vi "SV Measure Delay (Equal Polarity).vi"(0 "reference signal":waveform(dbl), 1 "ignore time stamp (T)":bool=TRUE, 5 "delayed signal":waveform(dbl), 7 "method":u16(ring)=1 items=["Trigger", "Cross correlation", "Phase lag"], 11 "error in":errorcluster, 12 "trigger parameters":T1={"level"=0.0, "slope"=0, "hysteresis"=-0.1} {"hysteresis" format="%.2p"; "slope" items=["Falling", "Rising"]; "level" format="%.2p"}) -> (4 "delay [s]":dbl format="%_4p", 6 "delay [samples]":dbl format="%_4f", 15 "error out":errorcluster)   [LabVIEW 2017, in "SoundVib_Calibration.lvlib"]
doc: "Use this VI to measure the propagation delay of a response signal. Use this VI when performing stimulus-response measurements to polarity normalize and time align the response signals prior to precision block processing. Use the equal polarity instance when the delayed signal exhibits equal polarity and simple time delay."
uses:
  <vilib>/addons/Sound and Vibration/svt_Calibration/SoundVib_Calibration.lvlib
  <vilib>/addons/_NISVFA/_Shared subVIs/Controls/svc_Analog Level Trigger Configuration.ctl
  <vilib>/Analysis/baseanly.llb/Mean (DBL).vi
  <vilib>/measure/matone.llb/Extract Single Tone Information 1 Chan.vi
  <vilib>/Analysis/2dsp.llb/1D Cross Correlation (DBL).vi
  <vilib>/measure/mamon.llb/Trigger Detection for 1 Channel.vi
  <vilib>/Analysis/NI_AALPro.lvlib
  <vilib>/measure/NI_MAPro.lvlib
  <vilib>/Analysis/NI_AAL_SigProc.lvlib
  <vilib>/Analysis/NI_AALBase.lvlib
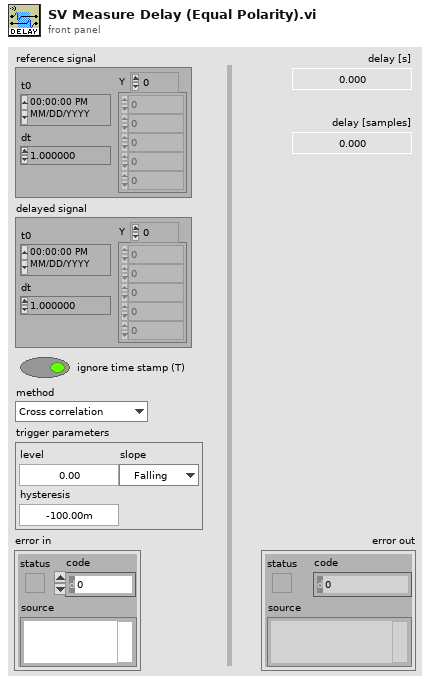
[diagram p1: front panel]
types:
  T1 = typedef "svc_Analog Level Trigger Configuration.ctl" = cluster{"level":dbl, "slope":u16, "hysteresis":dbl}
  T2 = cluster{"approx freq. (optional)":dbl, "search (+/- % of Fsampl.)":dbl}
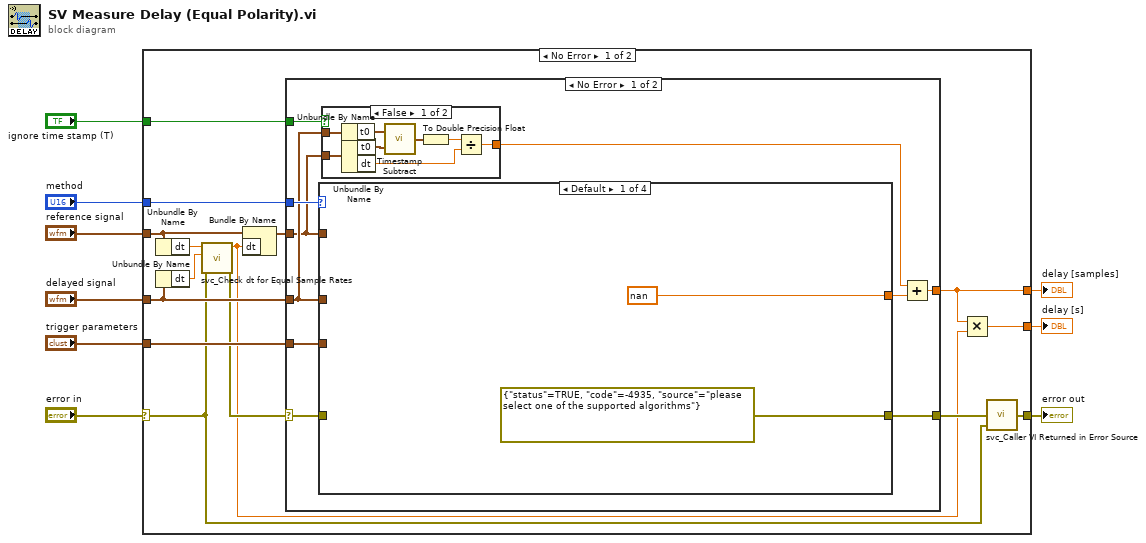
[diagram p0: block diagram]
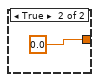
[diagram p2: hidden frame]
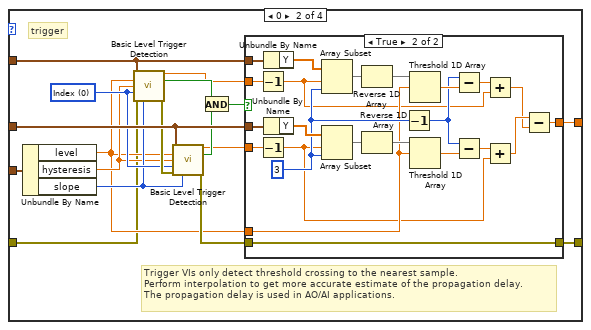
[diagram p3: hidden frame]
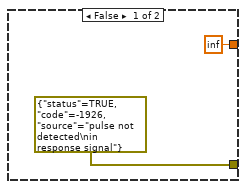
[diagram p4: hidden frame]
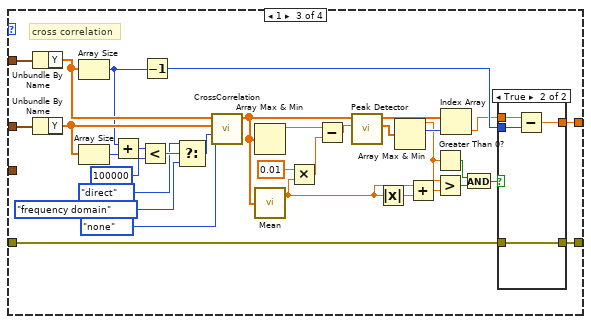
[diagram p5: hidden frame]
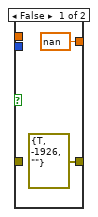
[diagram p6: hidden frame]
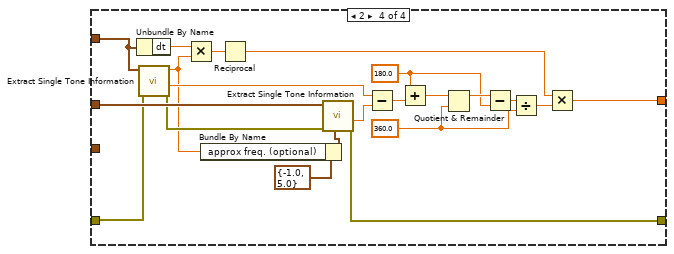
[diagram p7: hidden frame]
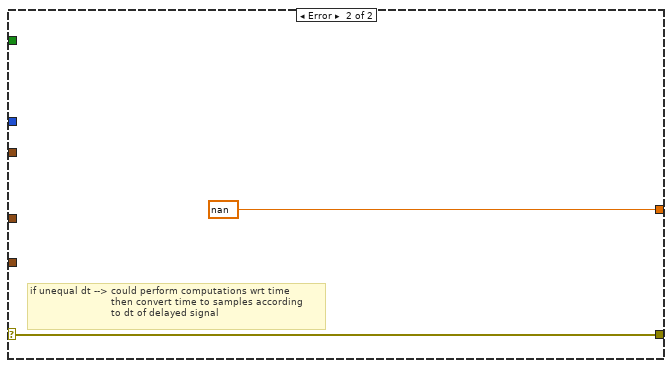
[diagram p8: hidden frame]
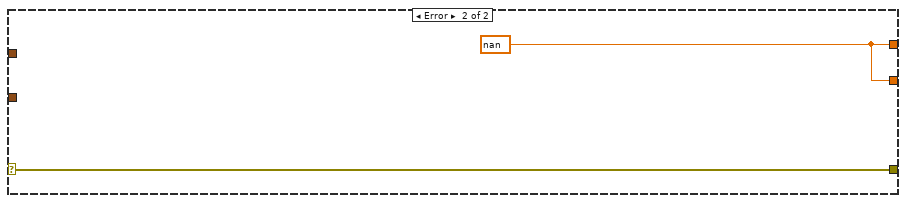
[diagram p9: hidden frame]
diagram:
  n1 = case shown="No Error" "error in" {
    selector: "error in" -> [w16 w151]
    tunnel: "method" -> [w24 _]
    tunnel: "trigger parameters" -> [w23 _]
    tunnel: [w17 w151] -> w7
    tunnel: "delayed signal" -> [w20 _]
    tunnel: "reference signal" -> [w14 _]
    tunnel: "ignore time stamp (T)" -> [w21 _]
    tunnel: [w12 w150] -> w3
    tunnel: [w10 w150] -> w1
    frame No Error {
      n2 = Unbundle By Name(w14) -> ("dt"=w19:dbl)
      n3 = Unbundle By Name(w20) -> ("dt"=w18:dbl)
      n4 = call <vilib>:"svc_Check dt for Equal Sample Rates.vi"("error in (no error)"=w16, "dt Y"=w18, "dt X"=w19) -> ("error out"=w15:errorcluster, "dt Y"=w11:dbl)  [unwired: 7 in]
      n5 = Bundle By Name(cluster=w14, "dt"=w11) -> (w13:waveform(dbl))
      n6 = case shown="No Error" w15 {
        selector: w15 -> [w26 w149]
        tunnel: w24 -> [w34 _]
        tunnel: w23 -> [w33 _]
        tunnel: [w32 w149] -> w22
        tunnel: w21 -> [w31 _]
        tunnel: [w30 nan] -> w12
        tunnel: w20 -> [w27 _]
        tunnel: w13 -> [w25 _]
        frame No Error {
          n7 = case shown="Default" w34 {
            tunnel: w27 -> [_ w62 w98 w147]
            tunnel: w25 -> [_ w61 w100 w140]
            tunnel: [nan w60 w117 w135] -> w29
            tunnel: w33 -> [_ w51 _ _]
            tunnel: w26 -> [_ w47 w101 w146]
            tunnel: [errorcluster {"status"=TRUE, "code"=-4935, "source"="please select one of the supported algorithms"} ("error out") w46 w115 w131] -> w32
            frame Default {
            }
            frame 0 {
              w52 = u16 0 items=["Index", "Time"] ("mode")
              # "trigger"
              # "Trigger VIs only detect threshold crossing to the nearest sample. \nPerform interpolation to get more accurate estimate of the propagation delay.\nThe propagation delay is used in AO/AI applications."
              n8 = Unbundle By Name(w51) -> ("level"=w48:dbl, "hysteresis"=w49:dbl, "slope"=w50:u16)
              n9 = call-poly <vilib>:"Basic Level Trigger Detection.vi"("signal in"=w61, "level"=w48, "hysteresis"=w49, "location mode"=w52, "error in (no error)"=w47, "trigger slope"=w50) -> ("trigger location"=w54:dbl, "trigger detected?"=w59:bool, "error out"=w57:errorcluster)  [unwired: 7 in]
              n10 = call-poly <vilib>:"Basic Level Trigger Detection.vi"("signal in"=w62, "level"=w48, "hysteresis"=w49, "location mode"=w52, "error in (no error)"=w57, "trigger slope"=w50) -> ("trigger location"=w55:dbl, "trigger detected?"=w58:bool, "error out"=w56:errorcluster)  [unwired: 7 in]
              n11 = And(x=w59, y=w58) -> (x .and. y?=w53:bool)
              n12 = case shown="True" w53 {
                tunnel: w55 -> [_ w72]
                tunnel: w54 -> [_ w84]
                tunnel: [inf w87] -> w60
                tunnel: w56 -> [_ w86]
                tunnel: [errorcluster {"status"=TRUE, "code"=-1926, "source"="pulse not detected\nin response signal"} ("error out") w86] -> w46
                tunnel: w61 -> [_ w85]
                tunnel: w48 -> [_ w71]
                tunnel: w62 -> [_ w76]
                frame False {
                }
                frame True {
                  w73 = 3 ("length")
                  n13 = Decrement(x=w84) -> (x-1=w68:dbl)
                  n14 = Decrement(x=w72) -> (x-1=w67:dbl)
                  n15 = Unbundle By Name(w85) -> ("Y"=w83:dbl[])
                  n16 = Unbundle By Name(w76) -> ("Y"=w75:dbl[])
                  n17 = Array Subset(array=w83, index=w68, length=w73) -> (w82:dbl[])
                  n18 = Array Subset(array=w75, index=w67, length=w73) -> (w77:dbl[])
                  n19 = Reverse 1D Array(array=w82) -> (reversed array=w81:dbl[])
                  n20 = Reverse 1D Array(array=w77) -> (reversed array=w78:dbl[])
                  n21 = Decrement(x=w73) -> (x-1=w74:i32)
                  n22 = Threshold 1D Array(2:w71, 3:w81) -> (0:w80:dbl)  [unwired: 1 in]
                  n23 = Threshold 1D Array(2:w71, 3:w78) -> (0:w79:dbl)  [unwired: 1 in]
                  n24 = Subtract(x=w74, y=w80) -> (x-y=w69:dbl)
                  n25 = Subtract(x=w74, y=w79) -> (x-y=w70:dbl)
                  n26 = Add(x=w69, y=w68) -> (x+y=w65:dbl)
                  n27 = Add(x=w70, y=w67) -> (x+y=w66:dbl)
                  n28 = Subtract(x=w66, y=w65) -> (x-y=w87:dbl)
                }
              }
            }
            frame 1 {
              # "cross correlation"
              n29 = Unbundle By Name(w100) -> ("Y"=w99:dbl[])
              n30 = Unbundle By Name(w98) -> ("Y"=w97:dbl[])
              n31 = Array Size(array=w99) -> (size(s)=w96:i32)
              n32 = Array Size(array=w97) -> (size(s)=w95:i32)
              n33 = Add(x=w96, y=w95) -> (x+y=w94:i32)
              n34 = Less?(x=w94, y=100000) -> (x < y?=w92:bool)
              n35 = Decrement(x=w96) -> (x-1=w116:i32)
              n36 = Select(t=enum32{"direct", "frequency domain"}."direct" ("algorithm"), s=w92, f=enum32{"direct", "frequency domain"}."frequency domain" ("algorithm")) -> (s? t:f=w89:enum32{"direct", "frequency domain"})
              n37 = call-poly <vilib>:"CrossCorrelation.vi"("normalization"=enum32{"none", "unbiased", "biased"}."none", "algorithm"=w89, "Y"=w97, "X"=w99) -> ("Rxy"=w111:dbl[])  [unwired: 6 in, 1 out]
              n38 = Array Max & Min(array=w111) -> (max value=w120:dbl)  [unwired: 3 out]
              n39 = call-poly <vilib>:"Mean.vi"("X"=w111) -> ("mean"=w104:dbl)  [unwired: 1 out]
              n40 = Multiply(x=0.01, y=w104) -> (x*y=w103:dbl)
              n41 = Subtract(x=w120, y=w103) -> (x-y=w119:dbl)
              n42 = call <vilib>:"Peak Detector.vi"("threshold"=w119, "X"=w111) -> ("Amplitudes"=w118:dbl[], "Locations"=w114:dbl[])  [unwired: 5 in, 3 out]
              n43 = Absolute Value(x=w104) -> (abs(x)=w109:dbl)
              n44 = Array Max & Min(array=w118) -> (max value=w106:dbl, max index (indices)=w113:i32)  [unwired: 2 out]
              n45 = Add(x=w104, y=w109) -> (x+y=w110:dbl)
              n46 = Greater Than 0?(x=w106) -> (x > 0?=w105:bool)
              n47 = Greater?(x=w106, y=w110) -> (0:w107:bool)
              n48 = Index Array(array=w114, index=w113) -> (element=w112:dbl)
              n49 = And(x=w105, y=w107) -> (x .and. y?=w108:bool)
              n50 = case shown="True" w108 {
                tunnel: [nan w126] -> w117
                tunnel: w116 -> [_ w125]
                tunnel: w101 -> [_ w124]
                tunnel: [errorcluster {"status"=TRUE, "code"=-1926, "source"=""} ("error out") w124] -> w115
                tunnel: w112 -> [_ w123]
                frame False {
                }
                frame True {
                  n51 = Subtract(x=w123, y=w125) -> (x-y=w126:dbl)
                }
              }
            }
            frame 2 {
              w127 = 180.0 ("y")
              w133 = 360.0 ("y")
              n52 = Unbundle By Name(w140) -> ("dt"=w139:dbl)
              n53 = call-poly <vilib>:"Extract Single Tone Information.vi"("error in (no error)"=w146, "time signal in"=w140) -> ("error out"=w145:errorcluster, "detected phase (deg)"=w142:dbl, "detected frequency"=w138:dbl)  [unwired: 4 in, 3 out]
              n54 = Multiply(x=w139, y=w138) -> (x*y=w136:dbl)
              n55 = Bundle By Name(cluster=T2 {"approx freq. (optional)"=-1.0, "search (+/- % of Fsampl.)"=5.0} ("advanced search"), "approx freq. (optional)"=w138) -> (w143:T2)
              n56 = Reciprocal(x=w136) -> (1/x=w132:dbl)
              n57 = call-poly <vilib>:"Extract Single Tone Information.vi"("advanced search"=w143, "error in (no error)"=w145, "time signal in"=w147) -> ("error out"=w131:errorcluster, "detected phase (deg)"=w141:dbl)  [unwired: 3 in, 4 out]
              n58 = Subtract(x=w142, y=w141) -> (x-y=w128:dbl)
              n59 = Add(x=w127, y=w128) -> (x+y=w130:dbl)
              n60 = Quotient & Remainder(x=w130, y=w133) -> (x-y*floor(x/y)=w137:dbl)  [unwired: 1 out]
              n61 = Subtract(x=w137, y=w127) -> (x-y=w129:dbl)
              n62 = Divide(x=w129, y=w133) -> (x/y=w134:dbl)
              n63 = Multiply(x=w132, y=w134) -> (x*y=w135:dbl)
            }
          }
          n64 = case shown="False" w31 {
            tunnel: w27 -> [w42 _]
            tunnel: w25 -> [w41 _]
            tunnel: [w36 0.0] -> w28
            frame False {
              n65 = Unbundle By Name(w42) -> ("t0"=w40:timestamp)
              n66 = Unbundle By Name(w41) -> ("t0"=w39:timestamp, "dt"=w35:dbl)
              n67 = call <vilib>:"Timestamp Subtract.vi"("y"=w39, "x"=w40) -> ("x - y"=w38:timestamp)
              n68 = To Double Precision Float(number=w38) -> (double precision float=w37:dbl)
              n69 = Divide(x=w37, y=w35) -> (x/y=w36:dbl)
            }
            frame True {
            }
          }
          n70 = Add(x=w28, y=w29) -> (x+y=w30:dbl)
        }
        frame Error {
          # "if unequal dt --> could perform computations wrt time \n                           then convert time to samples according\n                           to dt of delayed signal"
        }
      }
      n71 = Multiply(x=w12, y=w11) -> (x*y=w10:dbl)
      n72 = call <vilib>:"svc_Caller VI Returned in Error Source.vi"("warning input to caller"=w16, "error in (no error)"=w22) -> ("error out"=w17:errorcluster)  [unwired: 3 in]
    }
    frame Error {
      w150 = nan
    }
  }
  "delay [samples]" <- w3
  "error out" <- w7
  "delay [s]" <- w1
